vi "Initialize-Standard.vi"(5 "Reset? (F: No)":bool, 6 "Checksum (Disabled)":bool, 7 "ID Query? (Enabled)":bool=TRUE, 8 "error in (no error)":errorcluster, 9 "Serial Configuration (19200 : 19200 Baud)":u32(ring)=19200 items=["19200"=19200, "57600"=57600, "115200"=115200, "250000"=250000, "500000"=500000, "750000"=750000], 10 "Protocol (2: SCIP 2.0)":u32(ring)=2 items=["Convert to Latest", "SCIP 1.1", "SCIP 2.0"], 11 "VISA resource name":refnum<visa-resource-name>) -> (0 "error out":errorcluster, 3 "VISA resource name out":refnum<visa-resource-name>)   [LabVIEW 2011, in "Hokuyo URG Series.lvlib"]
doc: "Establishes communication with the instrument. It also places the instrument in a default state needed for other instrument driver operations. Therefore, call this VI before calling other instrument driver VIs for this instrument. Generally, you need to call the Initialize VI only once at the beginning of an application."
uses:
  Hokuyo URG Series.lvlib
panel:
  # "(c) 2009 National Instruments.  ALL RIGHTS RESERVED."
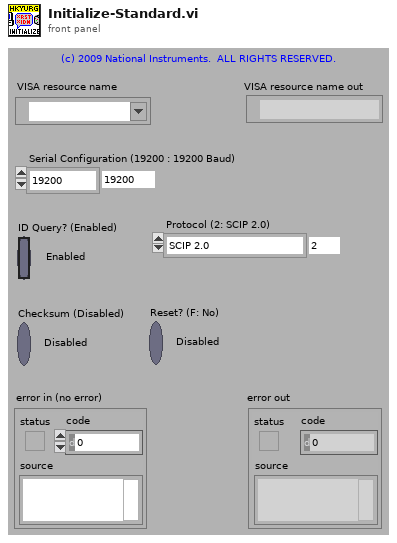
[diagram p1: front panel]
types:
  T1 = cluster{"Sensor Model":string, "Minimum Measurement":string, "Maximum Measurement":string, "Total Steps in Range":string, "First Step in Range":string, "Last Step in Range":string, "Front Step":string, "Standard Motor Speed":string}
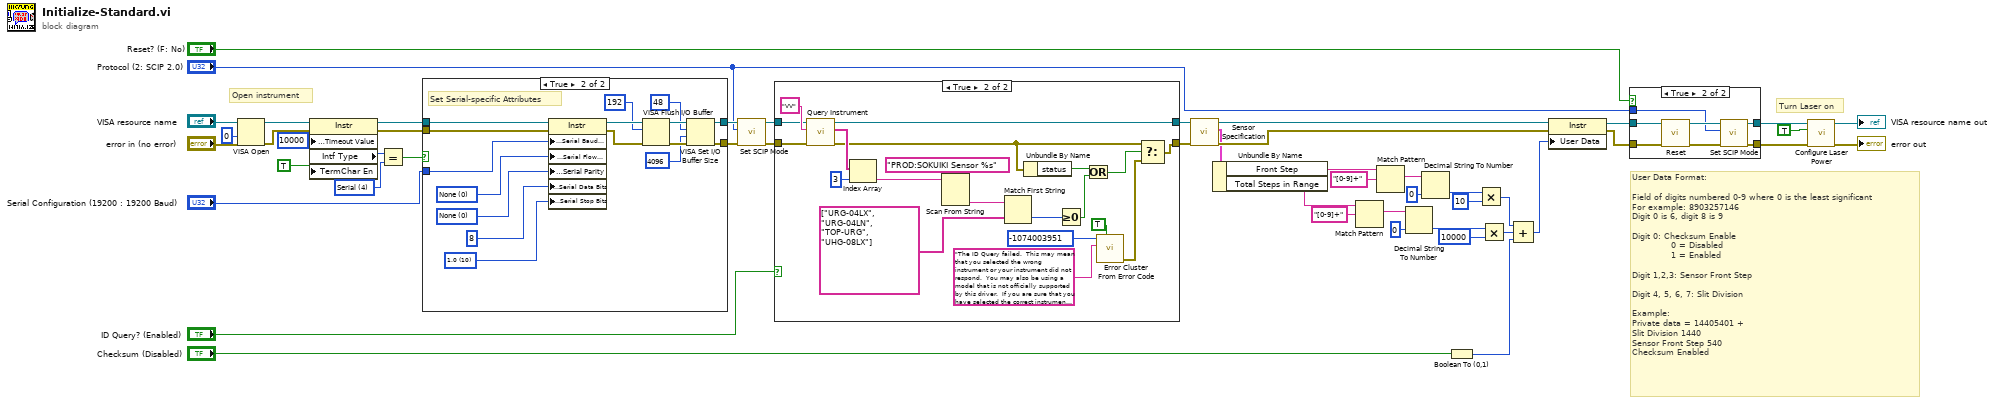
[diagram p0: block diagram]
diagram:
  w1 = u16 4 items=["GPIB"=1, "VXI"=2, "GPIB-VXI"=3, "Serial"=4, "PXI"=5, "TCPIP"=6, "USB"=7, "FireWire"=9] ("Interface Information:Interface Type")
  # "Open instrument"
  # "User Data Format:\n\nField of digits numbered 0-9 where 0 is the least significant\nFor example: 8903257146\nDigit 0 is 6, digit 8 is 9\n\nDigit 0: Checksum Enable\n             0 = Disabled\n             1 = Enabled\n\nDigit 1,2,3: Sensor Front Step\n\nDigit 4, 5, 6, 7: Slit Division\n\nExample:\nPrivate data = 14405401 +\nSlit Division 1440\nSensor Front Step 540\nChecksum Enabled"
  # "Turn Laser on"
  n1 = VISA Open(access mode=u32 0, error in (no error)="error in (no error)", VISA resource name="VISA resource name") -> (VISA resource name=w13:refnum<visa-resource-name>, error out=w12:errorcluster)  [unwired: 2 out]
  n2 = property class="Instr"(reference=w13, error in=w12, "General Settings:Timeout Value"=u32 10000, "TermChar En"=TRUE) -> (reference out=w48:refnum<visa-resource-name>, error out=w47:errorcluster, "Intf Type"=w2:u16)
  n3 = Equal?(x=w2, y=w1) -> (x = y?=w3:bool)
  n4 = case shown="True" w3 {
    tunnel: w48 -> [w51 w67]
    tunnel: w47 -> [w50 w66]
    tunnel: "Serial Configuration (19200 : 19200 Baud)" -> [_ w65]
    tunnel: [w50 w53] -> w40
    tunnel: [w51 w52] -> w39
    frame False {
    }
    frame True {
      w54 = u16 10 items=["1.0"=10, "1.5"=15, "2.0"=20] ("Serial Settings:Stop Bits")
      w56 = u16 0 items=["None", "Odd", "Even", "Mark", "Space"] ("Serial Settings:Parity")
      w57 = u16 0 items=["None", "XON/XOFF", "RTS/CTS", "XON/XOFF & RTS/CTS", "DTR/DSR", "XON/XOFF & DTR/DSR"] ("Serial Settings:Flow Control")
      # "Set Serial-specific Attributes"
      n5 = property class="Instr"(reference=w67, error in=w66, "Serial Settings:Serial Baud Rate"=w65, "Serial Settings:Serial Flow Control"=w57, "Serial Settings:Serial Parity"=w56, "Serial Settings:Serial Data Bits"=u16 8 ("Serial Settings:Data Bits"), "Serial Settings:Serial Stop Bits"=w54) -> (reference out=w61:refnum<visa-resource-name>, error out=w63:errorcluster)
      n6 = VISA Flush I/O Buffer(VISA resource name=w61, mask (16)=u16 192, error in (no error)=w63) -> (VISA resource name out=w64:refnum<visa-resource-name>, error out=w62:errorcluster)
      n7 = VISA Set I/O Buffer Size(VISA resource name=w64, mask (16)=u16 48, size (4096)=u32 4096 ("size (0)"), error in (no error)=w62) -> (VISA resource name out=w52:refnum<visa-resource-name>, error out=w53:errorcluster)
    }
  }
  n8 = call "Set SCIP Mode.vi"("error in (no error)"=w40, "Protocol (2: SCIP 2.0)"="Protocol (2: SCIP 2.0)", "VISA resource name"=w39) -> ("error out"=w37:errorcluster, "VISA resource name out"=w38:refnum<visa-resource-name>)  [unwired: 7 in]
  n9 = case shown="True" "ID Query? (Enabled)" {
    tunnel: w38 -> [w69 w75]
    tunnel: w37 -> [w68 w74]
    tunnel: [w69 w72] -> w34
    tunnel: [w68 w71] -> w32
    frame False {
    }
    frame True {
      n10 = call "Query Instrument.vi"("error in"=w74, "Command"="VV", "VISA Resource Name"=w75) -> ("error out"=w73:errorcluster, "Response Strings"=w77:string[], "VISA Resource Name Out"=w72:refnum<visa-resource-name>)  [unwired: 6 in]
      n11 = Index Array(array=w77, index=3) -> (element=w76:string)
      n12 = Scan From String(format string="PROD:SOKUIKI Sensor %s", input string=w76) -> (output 1=w79:string)  [unwired: 3 in, 3 out]
      n13 = Match First String(2:string[] ["URG-04LX", "URG-04LN", "TOP-URG", "UHG-08LX"], 3:w79) -> (0:w85:i32)  [unwired: 1 out]
      n14 = Unbundle By Name(w73) -> ("status"=w84:bool)
      n15 = Greater Or Equal To 0?(x=w85) -> (x >= 0?=w83:bool)
      n16 = Or(x=w84, y=w83) -> (x .or. y?=w82:bool)
      n17 = call <vilib>:"Error Cluster From Error Code.vi"("show call chain? (False)"=TRUE, "error message (\"\")"="The ID Query failed.  This may mean that you selected the wrong instrument or your instrument did not respond.  You may also be using a model that is not officially supported by this driver.  If you are sure that you have selected the correct instrument and it is responding, try disabling the ID Query." ("Source (VI Name)"), "error code (0)"=-1074003951 ("Code")) -> ("error out"=w89:errorcluster)  [unwired: 1 in, 5 out]
      n18 = Select(t=w73, s=w82, f=w89) -> (s? t:f=w71:errorcluster)
    }
  }
  n19 = call "Sensor Specification.vi"("error in (no error)"=w32, "VISA resource name"=w34) -> ("error out"=w33:errorcluster, "Instrument Specifications"=w31:T1, "VISA resource name out"=w35:refnum<visa-resource-name>)  [unwired: 7 in]
  n20 = Unbundle By Name(w31) -> ("Front Step"=w20:string, "Total Steps in Range"=w16:string)
  n21 = Match Pattern(string=w16, regular expression="[0-9]+") -> (match substring=w15:string)  [unwired: 1 in, 3 out]
  n22 = Match Pattern(string=w20, regular expression="[0-9]+") -> (match substring=w18:string)  [unwired: 1 in, 3 out]
  n23 = Decimal String To Number(string=w15, default (0L)=u32 0 ("default (0 I32)")) -> (number=w27:u32)  [unwired: 1 in, 1 out]
  n24 = Decimal String To Number(string=w18, default (0L)=u32 0 ("default (0 I32)")) -> (number=w28:u32)  [unwired: 1 in, 1 out]
  n25 = Boolean To (0,1)(Boolean="Checksum (Disabled)") -> (0, 1=w24:i16)
  n26 = Multiply(x=w28, y=u32 10) -> (x*y=w22:u32)
  n27 = Multiply(x=w27, y=u32 10000) -> (x*y=w23:u32)
  n28 = Compound Arithmetic op=ADD(w22, w23, w24) -> (w21:u32)
  n29 = property class="Instr"(reference=w35, error in=w33, "User Data"=w21) -> (reference out=w9:refnum<visa-resource-name>, error out=w7:errorcluster)
  n30 = case shown="True" "Reset? (F: No)" {
    tunnel: w9 -> [w91 w97]
    tunnel: w7 -> [w90 w98]
    tunnel: [w90 w93] -> w6
    tunnel: [w91 w95] -> w8
    tunnel: "Protocol (2: SCIP 2.0)" -> [_ w92]
    frame False {
    }
    frame True {
      n31 = call "Reset.vi"("error in (no error)"=w98, "VISA resource name"=w97) -> ("error out"=w94:errorcluster, "VISA resource name out"=w96:refnum<visa-resource-name>)  [unwired: 8 in]
      n32 = call "Set SCIP Mode.vi"("error in (no error)"=w94, "Protocol (2: SCIP 2.0)"=w92, "VISA resource name"=w96) -> ("error out"=w93:errorcluster, "VISA resource name out"=w95:refnum<visa-resource-name>)  [unwired: 7 in]
    }
  }
  n33 = call "Configure Laser Power.vi"("error in (no error)"=w6, "Laser Power"=TRUE ("Laser"), "VISA resource name"=w8) -> ("error out"=→"error out":errorcluster, "VISA resource name out"=→"VISA resource name out":refnum<visa-resource-name>)  [unwired: 7 in]
